vi "specu1a 1.0.0 Param Cluster to Param Enum.vi"(1 "Cluster in":T4) -> (0 "Parameters":T1={"Integration time"=10000, "Gain"=enum."No Function", "TriggerEdge"=enum."No Function", "Trigger Mode"=enum."Asynchronous", "Reserved"=0})   [LabVIEW 2019]
uses:
  Controls/specu1a 1.0.0 Parameters.ctl
  Controls/specu1a 1.0.0 Trigger Edge.ctl
  Controls/specu1a 1.0.0 Trigger Mode.ctl
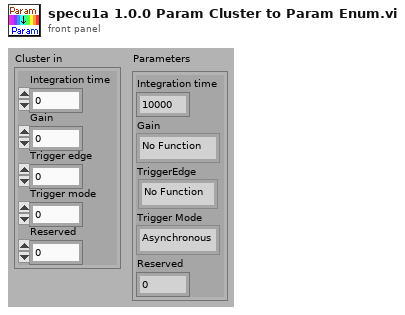
[diagram p1: front panel]
types:
  T1 = typedef "specu1a 1.0.0 Parameters.ctl" = cluster{"Integration time":u32, "Gain":enum16{"Low", "High", "No Function"}, "TriggerEdge":T2, "Trigger Mode":T3, "Reserved":u8}
  T2 = typedef "specu1a 1.0.0 Trigger Edge.ctl" = enum16{"Rising", "Falling", "No Function"}
  T3 = typedef "specu1a 1.0.0 Trigger Mode.ctl" = enum16{"Internal", "Asynchronous", "Synchronous"}
  T4 = cluster{"Integration time":u32, "Gain":u8, "Trigger edge":u8, "Trigger mode":u8, "Reserved":u8}
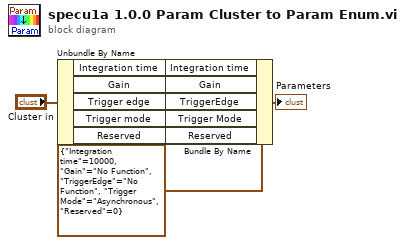
[diagram p0: block diagram]
diagram:
  n1 = Unbundle By Name("Cluster in") -> ("Integration time"=w1:u32, "Gain"=w6:u8, "Trigger edge"=w5:u8, "Trigger mode"=w4:u8, "Reserved"=w3:u8)
  n2 = Bundle By Name(cluster=T1 {"Integration time"=10000, "Gain"=enum."No Function", "TriggerEdge"=enum."No Function", "Trigger Mode"=enum."Asynchronous", "Reserved"=0} ("Parameters"), "Integration time"=w1, "Gain"=w6, "TriggerEdge"=w5, "Trigger Mode"=w4, "Reserved"=w3) -> (→"Parameters":T1)
